vi "Floating Keypad.vi"(8 "Position":cluster{"Top":i16, "Left":i16}, 9 "Length":i32=10, 10 "StringIn":string, 11 "Allow dot":bool) -> (2 "StringOut":string caption="Display")   [LabVIEW 2015]
panel:
  in  "Dot":bool
  in  "1":bool
  in  "Clear":bool
  in  "Back":bool
  in  "0":bool
  in  "9":bool
  in  "8":bool
  in  "7":bool
  in  "6":bool
  in  "5":bool
  in  "4":bool
  in  "3":bool
  in  "2":bool
  in  "stop":bool
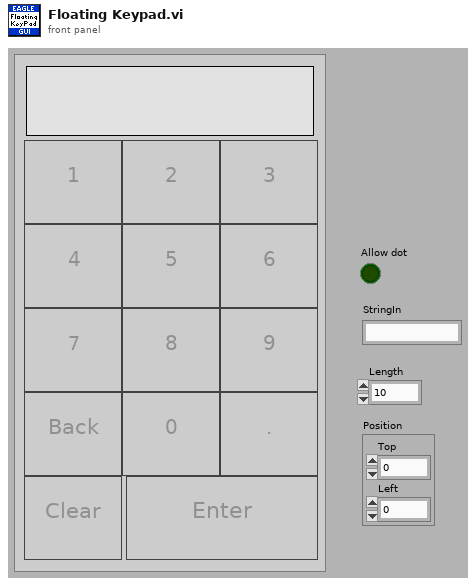
[diagram p1: front panel]
types:
  T1 = typedef "LVRectTypeDef.ctl" = cluster{"Left":i16, "Top":i16, "Right":i16, "Bottom":i16}
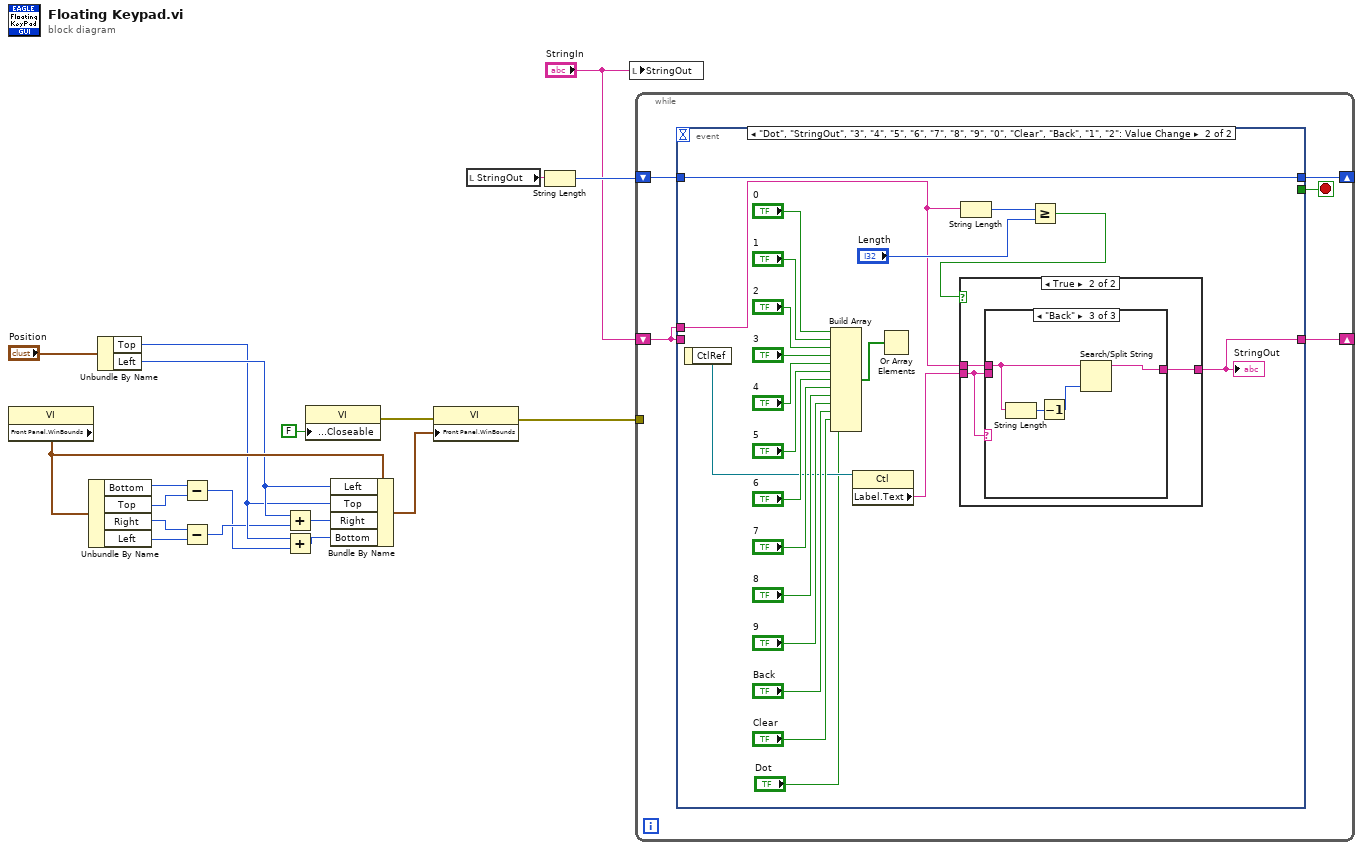
[diagram p0: block diagram]
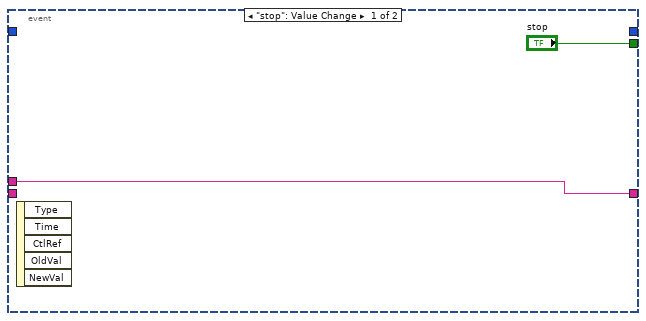
[diagram p2: hidden frame]
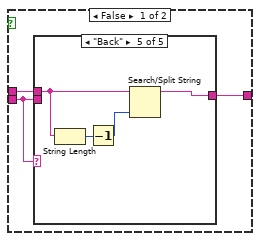
[diagram p3: hidden frame]
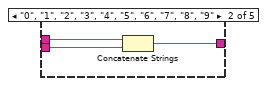
[diagram p5: hidden frame]
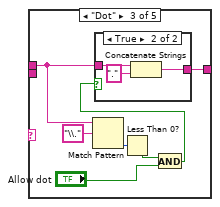
[diagram p6: hidden frame]
diagram:
  n1 = property class="VI"() -> ("Front Panel.WinBounds"=w16:T1)  [unwired: 2 in, 2 out]
  n2 = Unbundle By Name(w16) -> ("Bottom"=w8:i16, "Top"=w7:i16, "Right"=w6:i16, "Left"=w5:i16)
  n3 = Unbundle By Name("Position") -> ("Top"=w11:i16, "Left"=w13:i16)
  n4 = Subtract(x=w8, y=w7) -> (x-y=w3:i16)
  n5 = Subtract(x=w6, y=w5) -> (x-y=w4:i16)
  n6 = Add(x=w13, y=w4) -> (x+y=w14:i16)
  n7 = Add(x=w11, y=w3) -> (x+y=w12:i16)
  n8 = property class="VI"("Front Panel.Closeable"=FALSE ("Front Panel Window:Closeable")) -> (error out=w2:errorcluster)  [unwired: 2 in, 1 out]
  n9 = Bundle By Name(cluster=w16, "Left"=w13, "Top"=w11, "Right"=w14, "Bottom"=w12) -> (w10:T1)
  n10 = property class="VI"(error in=w2, "Front Panel.WinBounds"=w10) -> (error out=w9:errorcluster)  [unwired: 1 in, 1 out]
  n11 = local read "StringOut"() -> (w19:string)
  n12 = String Length(string=w19) -> (length=w18:i32)
  n13 = local write "StringOut"("StringIn") -> ()
  n14 = while {
    shift-right: [w24] -> _
    shift-left: "StringIn" -> [w22]
    shift-right: [w20] -> _
    shift-left: w18 -> [w21]
    tunnel: w9 -> [_]
    stop <- w23 stop-if-true
    n15 = event shown="[1] \"Dot\", \"StringOut\", \"3\", \"4\", \"5\", \"6\", \"7\", \"8\", \"9\", \"0\", \"Clear\", \"Back\", \"1\", \"2\": Value Change" {
      selector: _ -> [_ _]
      dyn-events: _ -> [_ _]
      timeout: _ -> [_ _]
      tunnel: [w26 w37] -> w24
      tunnel: w22 -> [w26 w28]
      tunnel: ["stop" _] -> w23
      tunnel: w22 -> [_ _]
      tunnel: w21 -> [_ w36]
      tunnel: [_ w36] -> w20
      event "stop": Value Change {
        n16 = event-data() -> ()  [unwired: 1 in, 5 out]
      }
      event "Dot", "StringOut", "3", "4", "5", "6", "7", "8", "9", "0", "Clear", "Back", "1", "2": Value Change {
        n17 = event-data() -> ("CtlRef"=w33:refnum<vi>)  [unwired: 1 in]
        n18 = Build Array("0", "1", "2", "3", "4", "5", "6", "7", "8", "9", "Back", "Clear", "Dot") -> (w38:bool[])
        n19 = property class="Ctl"(reference=w33) -> ("Label.Text"=w32:string)  [unwired: 1 in, 2 out]
        n20 = Or Array Elements(Boolean array=w38) -> ()  [unwired: 1 out]
        n21 = String Length(string=w28) -> (length=w30:i32)
        n22 = Greater Or Equal?(x=w30, y="Length") -> (x >= y?=w27:bool)
        n23 = case shown="True" w27 {
          tunnel: w28 -> [w51 w73]
          tunnel: [w50 w72] -> w37
          tunnel: w32 -> [w49 w71]
          frame False {
            n24 = case shown="\"Back\"" w49 {
              tunnel: w49 -> [_ w54 _ _ _]
              tunnel: w51 -> [w52 w55 w61 _ w70]
              tunnel: [w52 w53 w62 _ w67] -> w50
              frame Default {
              }
              frame "0", "1", "2", "3", "4", "5", "6", "7", "8", "9" {
                n25 = Concatenate Strings(w55, w54) -> (w53:string)
              }
              frame "Dot" {
                n26 = Match Pattern(string=w61, regular expression="\\.") -> (offset past match=w59:i32)  [unwired: 1 in, 3 out]
                n27 = Less Than 0?(x=w59) -> (x < 0?=w58:bool)
                n28 = And(x=w58, y="Allow dot") -> (x .and. y?=w56:bool)
                n29 = case shown="True" w56 {
                  tunnel: w61 -> [w63 w66]
                  tunnel: [w63 w65] -> w62
                  frame False {
                  }
                  frame True {
                    n30 = Concatenate Strings(w66, "." ("string")) -> (w65:string)
                  }
                }
              }
              frame "Clear" {
              }
              frame "Back" {
                n31 = String Length(string=w70) -> (length=w69:i32)
                n32 = Decrement(x=w69) -> (x-1=w68:i32)
                n33 = Search/Split String(string=w70, offset (0)=w68) -> (substring before match=w67:string)  [unwired: 1 in, 2 out]
              }
            }
          }
          frame True {
            n34 = case shown="\"Back\"" w71 {
              tunnel: w71 -> [_ _ _]
              tunnel: w73 -> [w74 _ w78]
              tunnel: [w74 _ w75] -> w72
              frame Default {
              }
              frame "Clear" {
              }
              frame "Back" {
                n35 = String Length(string=w78) -> (length=w77:i32)
                n36 = Decrement(x=w77) -> (x-1=w76:i32)
                n37 = Search/Split String(string=w78, offset (0)=w76) -> (substring before match=w75:string)  [unwired: 1 in, 2 out]
              }
            }
          }
        }
        "StringOut" <- w37
      }
    }
  }
